vi "CRIOUI.vi"() -> ()   [LabVIEW 2013, in "PLTarget cRIO.lvclass"]
uses:
  PLTarget cRIO.lvclass
  <vilib>/NI/Configuration Framework/Node/NodeRef.ctl
  <vilib>/NI/Configuration Framework/Node/NISE_CEF_Node.lvclass
  <vilib>/NI/AMC/Message Queue.ctl
  <vilib>/NI/AMC/Message.ctl
  <vilib>/NI/Tools/Keyed Array/KeyedArray.ctl
  <vilib>/NI/Configuration Framework/Node/UserEventRef.ctl
  <vilib>/NI/Configuration Framework/Controls/EventCluster.ctl
  <vilib>/NI/Tag Bus Module Framework/root configuration/Target Types.ctl
  PLTarget cRIO.lvclass/PLTarget cRIO.ctl
  Framework Configuration Classes/target configuration/PL_Target Configuration.lvclass/PL_Target Configuration.ctl
  Configuration Editor/Classes/Targets/Targets.lvclass/Targets.ctl
  <vilib>/NI/AMC/Create Single Message.vi
  <vilib>/NI/AMC/Update Message Routing Info.vi
  <vilib>/NI/Configuration Framework/serializable configuration/get alias.vi
  <vilib>/NI/Configuration Framework/serializable configuration/set alias.vi
  <vilib>/NI/AMC/Send Message.vi
  <vilib>/NI/AMC/AMC.lvlib
  Framework Configuration Classes/target configuration/PL_Target Configuration.lvclass
  Configuration Editor/Classes/Targets/Targets.lvclass
  <vilib>/NI/Tools/Keyed Array/Tools_KeyedArray.lvlib
  <vilib>/NI/Configuration Framework/NISE_CEF_TreeControl.lvlib
  <vilib>/NI/Tag Bus Module Framework/root configuration/TBM configuration.lvclass
panel:
  in  "Local Bitfile Path":path
  in  "load bitfile":bool
  in  "bitfile path on target relative to root (c:\\ or /home/lvuser/)":path
  in  "RIO FPGA":string="RIO0"
  in  "Target Type":T1=enum."Linux RT ARM"
  in  "path to deploy on target relative to root (c:\\ or /home/lvuser/)":path
  in  "IP":string
  in  "user event":T2
  in  "main queue":T3
  in  "Name":string
  in  "node ref":T4
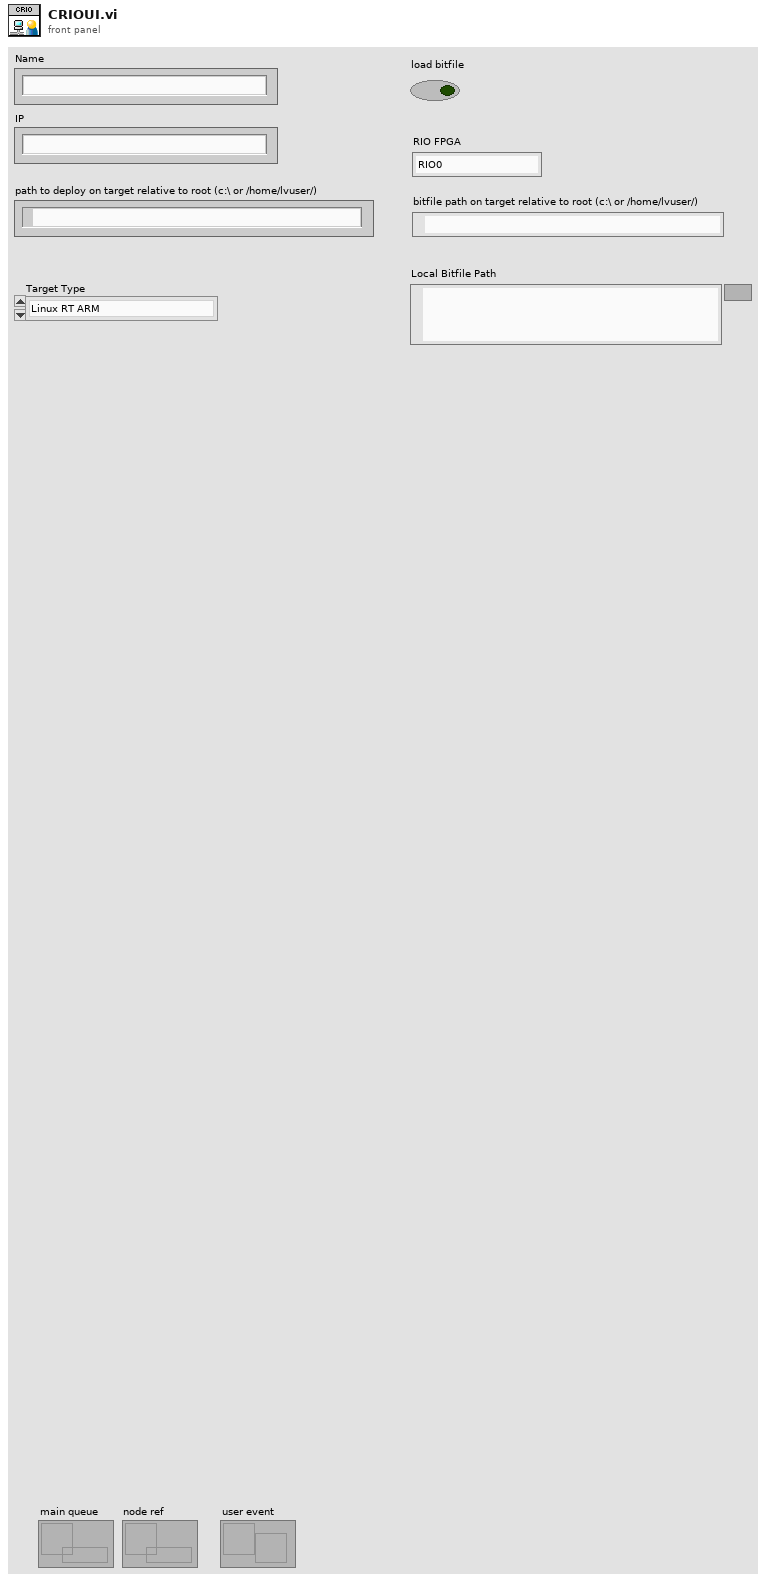
[diagram p1: front panel]
types:
  T1 = typedef "TBM configuration.lvclass/Target Types.ctl" = enum16{"Windows", "Mac", "Linux", "Linux RT ARM", "VxWorks", "Pharlap", "Other", "Linux RT x64"}
  T2 = typedef "NISE_CEF_Node.lvclass/UserEventRef.ctl" = refnum<user-event>
  T3 = typedef "AMC.lvlib/Message Queue.ctl" = refnum<queue>
  T4 = typedef "NISE_CEF_Node.lvclass/NodeRef.ctl" = refnum<data-value>
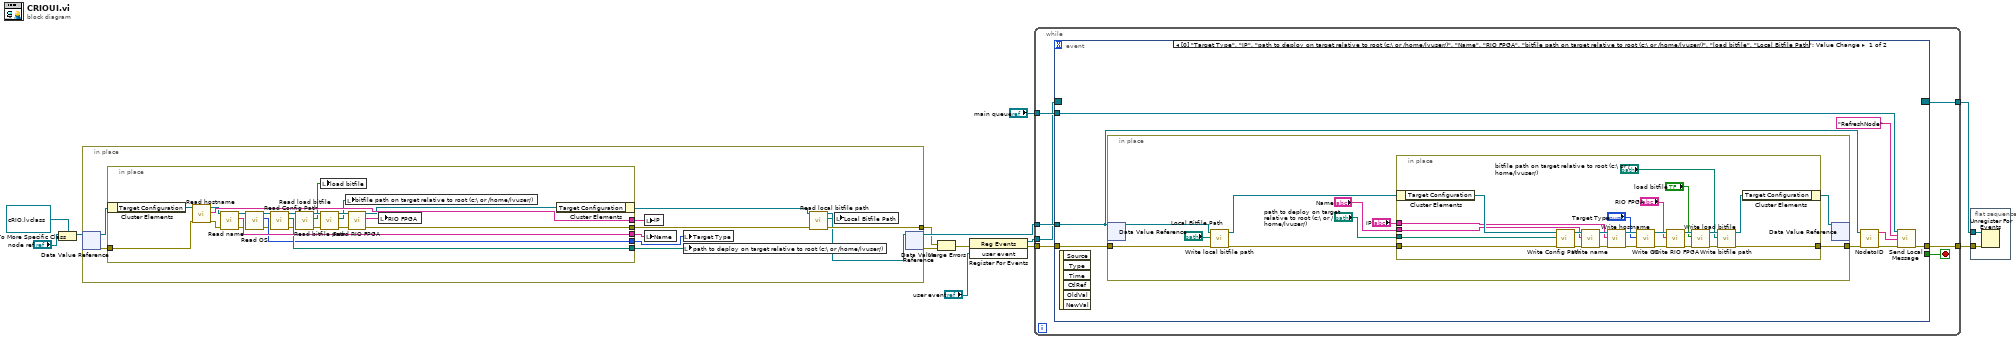
[diagram p0: block diagram]
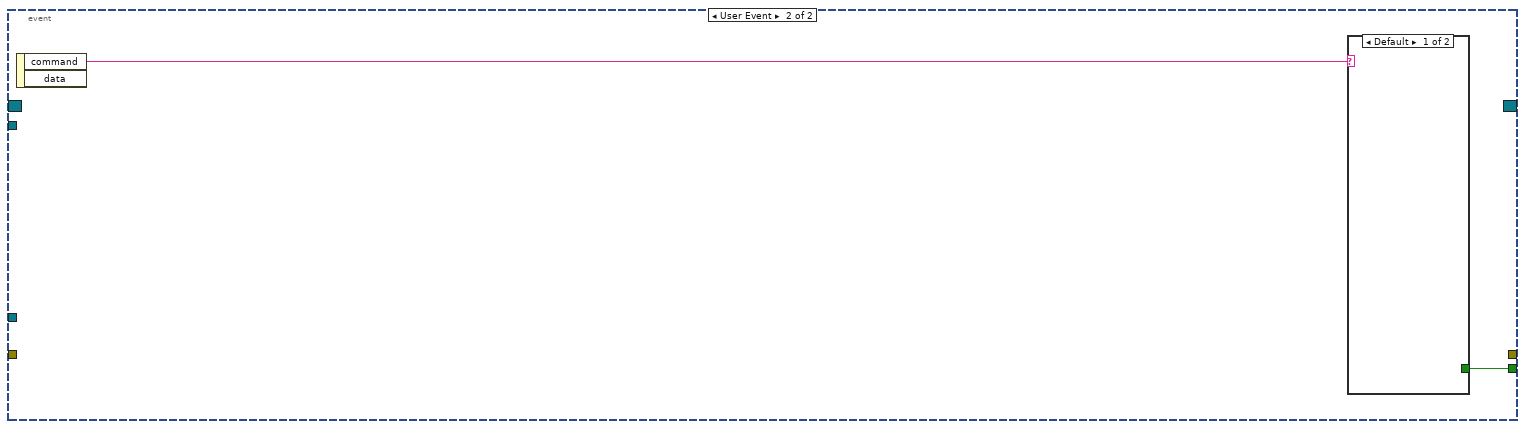
[diagram p2: hidden frame]
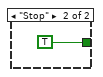
[diagram p3: hidden frame]
diagram:
  n1 = To More Specific Class(target class=refnum<data-value> refnum ("data value reference"), reference="node ref") -> (specific class reference=w5:refnum<data-value>)  [unwired: 1 in, 1 out]
  n2 = in-place {
    in-place-border: [w17] -> w3
    n3 = in-place-dvr #1(w5) -> (w21:refnum<class "PLTarget cRIO.lvclass">, w19:errorcluster)
    n4 = in-place {
      in-place-border: [w47] -> w24
      in-place-border: [w42] -> w22
      in-place-border: [w46] -> w23
      in-place-border: [w40] -> w20
      in-place-border: w19 -> [w29]
      in-place-border: [w28] -> w18
      n5 = in-place-cluster #2(w21) -> ("Target Configuration"=w43:refnum<class "PL_Target Configuration.lvclass">)
      n6 = call "Read hostname.vi"("error in"=w29, "PL_Target Configuration in"=w43) -> ("error out"=w39:errorcluster, "hostname"=w46:string, "PL_Target Configuration out"=w44:refnum<class "PL_Target Configuration.lvclass">)  [unwired: 7 in]
      n7 = call "Read name.vi"("error in"=w39, "PL_Local Target Configuration in"=w44) -> ("error out"=w38:errorcluster, "name"=w47:string, "PL_Local Target Configuration out"=w45:refnum<class "PL_Target Configuration.lvclass">)  [unwired: 7 in]
      n8 = call "Read OS.vi"("error in"=w38, "PL_Target Configuration in"=w45) -> ("error out"=w37:errorcluster, "Target Types"=w40:T1, "PL_Target Configuration out"=w41:refnum<class "PL_Target Configuration.lvclass">)  [unwired: 7 in]
      n9 = call "Read Config Path.vi"("error in"=w37, "PL_Local Target Configuration in"=w41) -> ("error out"=w30:errorcluster, "Config Path"=w42:path, "PL_Local Target Configuration out"=w31:refnum<class "PL_Target Configuration.lvclass">)  [unwired: 7 in]
      n10 = call "Read load bitfile.vi"("error in"=w30, "PL_Target Configuration in"=w31) -> ("error out"=w34:errorcluster, "load bitfile"=w25:bool, "PL_Target Configuration out"=w33:refnum<class "PL_Target Configuration.lvclass">)  [unwired: 7 in]
      n11 = local write "load bitfile"(w25) -> ()
      n12 = call "Read bitfile path.vi"("error in"=w34, "PL_Target Configuration in"=w33) -> ("error out"=w36:errorcluster, "bitfile path"=w26:path, "PL_Target Configuration out"=w35:refnum<class "PL_Target Configuration.lvclass">)  [unwired: 7 in]
      n13 = local write "bitfile path on target relative to root (c:\\ or /home/lvuser/)"(w26) -> ()
      n14 = call "Read RIO FPGA.vi"("error in"=w36, "PL_Target Configuration in"=w35) -> ("error out"=w28:errorcluster, "RIO FPGA"=w27:string, "PL_Target Configuration out"=w32:refnum<class "PL_Target Configuration.lvclass">)  [unwired: 7 in]
      n15 = local write "RIO FPGA"(w27) -> ()
      n16 = in-place-cluster #2("Target Configuration"=w32) -> (w15:refnum<class "PLTarget cRIO.lvclass">)
    }
    n17 = local write "IP"(w23) -> ()
    n18 = local write "Name"(w24) -> ()
    n19 = local write "Target Type"(w20) -> ()
    n20 = local write "path to deploy on target relative to root (c:\\ or /home/lvuser/)"(w22) -> ()
    n21 = call "Read local bitfile path.vi"("error in"=w18, "Targets in"=w15) -> ("error out"=w17:errorcluster, "bitfile path"=w14:path, "Targets out"=w16:refnum<class "PLTarget cRIO.lvclass">)  [unwired: 7 in]
    n22 = local write "Local Bitfile Path"(w14) -> ()
    n23 = in-place-dvr #1(w16) -> (w13:refnum<data-value>, w1:errorcluster)
  }
  n24 = Merge Errors(w3, w1) -> (w2:errorcluster)
  n25 = register-events(error in=w2, "user event") -> (reference out=w10:refnum<event-registration>, error out=w7:errorcluster)  [unwired: 1 in]
  n26 = while {
    tunnel: w13 -> [w54]
    tunnel: "main queue" -> [w53]
    tunnel: w10 -> [w52]
    tunnel: [w51] -> w9
    tunnel: [w49] -> w8
    tunnel: w7 -> [w48]
    stop <- w50 stop-if-true
    n27 = event shown="[0] \"Target Type\", \"IP\", \"path to deploy on target relative to root (c:\\ or /home/lvuser/)\", \"Name\", \"RIO FPGA\", \"bitfile path on target relative to root (c:\\ or /home/lvuser/)\", \"load bitfile\", \"Local Bitfile Path\": Value Change" {
      selector: w52 -> [_ _]
      dyn-events: [_ _] -> w51
      timeout: _ -> [_ _]
      tunnel: w54 -> [w60 _]
      tunnel: w53 -> [w61 _]
      tunnel: [_ w96] -> w50
      tunnel: [w58 _] -> w49
      tunnel: w48 -> [w57 _]
      event "IP", "path to deploy on target relative to root (c:\\ or /home/lvuser/)", "Name", "RIO FPGA", "bitfile path on target relative to root (c:\\ or /home/lvuser/)", "load bitfile", "Local Bitfile Path": Value Change {
        n28 = event-data() -> ()  [unwired: 1 in, 6 out]
        n29 = in-place {
          in-place-border: w57 -> [w64]
          in-place-border: [w68] -> w56
          n30 = in-place-dvr #3(w60) -> (w67:refnum<class "PLTarget cRIO.lvclass">)  [unwired: 1 out]
          n31 = call "Write local bitfile path.vi"("error in"=w64, "bitfile path"="Local Bitfile Path", "Targets in"=w67) -> ("error out"=w65:errorcluster, "Targets out"=w66:refnum<class "PLTarget cRIO.lvclass">)  [unwired: 7 in]
          n32 = in-place {
            in-place-border: "path to deploy on target relative to root (c:\\ or /home/lvuser/)" -> [w94]
            in-place-border: "IP" -> [w91]
            in-place-border: "Name" -> [w90]
            in-place-border: w65 -> [w77]
            in-place-border: [w76] -> w68
            n33 = in-place-cluster #4(w66) -> ("Target Configuration"=w95:refnum<class "PL_Target Configuration.lvclass">)
            n34 = call "Write Config Path.vi"("error in"=w77, "Config Path"=w94, "PL_Local Target Configuration in"=w95) -> ("error out"=w81:errorcluster, "PL_Local Target Configuration out"=w93:refnum<class "PL_Target Configuration.lvclass">)  [unwired: 7 in]
            n35 = call "Write name.vi"("error in"=w81, "name"=w90, "PL_Local Target Configuration in"=w93) -> ("error out"=w80:errorcluster, "PL_Local Target Configuration out"=w92:refnum<class "PL_Target Configuration.lvclass">)  [unwired: 7 in]
            n36 = call "Write hostname.vi"("error in"=w80, "hostname"=w91, "PL_Target Configuration in"=w92) -> ("error out"=w79:errorcluster, "PL_Target Configuration out"=w89:refnum<class "PL_Target Configuration.lvclass">)  [unwired: 7 in]
            n37 = call "Write OS.vi"("error in"=w79, "Target Types"="Target Type", "PL_Target Configuration in"=w89) -> ("error out"=w78:errorcluster, "PL_Target Configuration out"=w83:refnum<class "PL_Target Configuration.lvclass">)  [unwired: 7 in]
            n38 = call "Write RIO FPGA.vi"("error in"=w78, "RIO FPGA"="RIO FPGA", "PL_Target Configuration in"=w83) -> ("error out"=w85:errorcluster, "PL_Target Configuration out"=w84:refnum<class "PL_Target Configuration.lvclass">)  [unwired: 7 in]
            n39 = call "Write load bitfile.vi"("error in"=w85, "load bitfile"="load bitfile", "PL_Target Configuration in"=w84) -> ("error out"=w87:errorcluster, "PL_Target Configuration out"=w86:refnum<class "PL_Target Configuration.lvclass">)  [unwired: 7 in]
            n40 = call "Write bitfile path.vi"("error in"=w87, "bitfile path"="bitfile path on target relative to root (c:\\ or /home/lvuser/)", "PL_Target Configuration in"=w86) -> ("error out"=w76:errorcluster, "PL_Target Configuration out"=w82:refnum<class "PL_Target Configuration.lvclass">)  [unwired: 7 in]
            n41 = in-place-cluster #4("Target Configuration"=w82) -> (w72:refnum<class "PLTarget cRIO.lvclass">)
          }
          n42 = in-place-dvr #3(w72) -> ()  [unwired: 2 out]
        }
        n43 = call <vilib>:"NodetoID.vi"("error in"=w56, "node ref"=w60) -> ("error out"=w55:errorcluster, "ID"=w59:string)  [unwired: 8 in]
        n44 = call <vilib>:"Send Local Message.vi"("message queue in"=w61, "message name"="RefreshNode" ("Message Name"), "message value"=w59, "error in"=w55) -> ("error out"=w58:errorcluster)  [unwired: 9 in, 2 out]
      }
      event User Event {
        n45 = event-data() -> ("command"=w97:string)  [unwired: 1 in, 1 out]
        n46 = case shown="Default" w97 {
          tunnel: [_ TRUE] -> w96
          frame Default {
          }
          frame "Stop" {
          }
        }
      }
    }
  }
  n47 = flat-sequence {
    tunnel: w9 -> [w100]
    tunnel: w8 -> [w99]
    frame #0 {
      n48 = Unregister For Events(event registration refnum=w100, error in=w99) -> ()  [unwired: 1 out]
    }
  }
